vi "Move In Direction.vi"(7 "move toward? (T)":bool=TRUE, 10 "direction options":T1[](array[typedef])=[enum."NW", enum."N", enum."NE", enum."E", enum."SE", enum."S", enum."SW", enum."W"], 11 "goal angle (deg)":dbl) -> (2 "ordered directions":T1[](array[typedef]), 3 "best direction":T1)   [LabVIEW 2020, in "DS Square.lvlib"]
uses:
  DS Square.lvlib
  Type Defs/Direction Enum.ctl
  <vilib>/Analysis/baseanly.llb/Real Dot Product.vi
  <vilib>/Analysis/NI_AALBase.lvlib
  Type Defs/SB Type Defs.lvlib
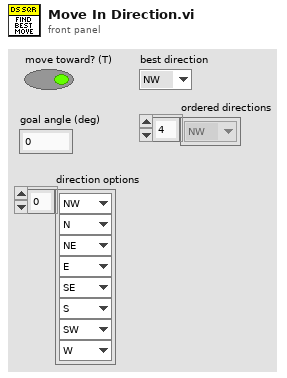
[diagram p1: front panel]
types:
  T1 = typedef "SB Type Defs.lvlib/Direction Enum.ctl" = enum16{"NW", "N", "NE", "E", "SE", "S", "SW", "W"}
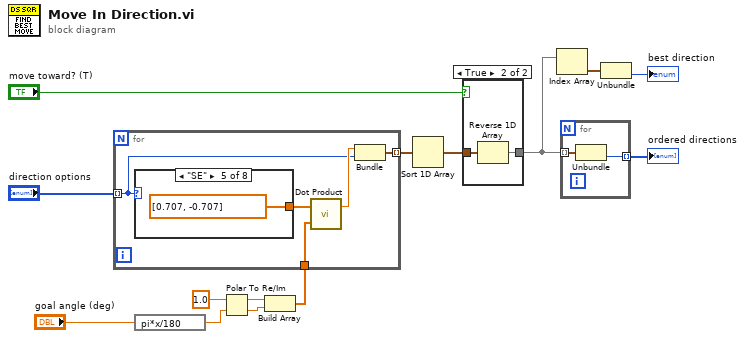
[diagram p0: block diagram]
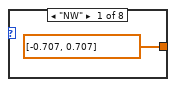
[diagram p3: hidden frame]
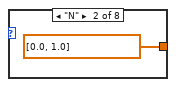
[diagram p4: hidden frame]
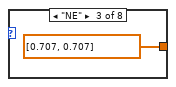
[diagram p5: hidden frame]
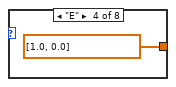
[diagram p6: hidden frame]
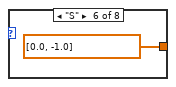
[diagram p7: hidden frame]
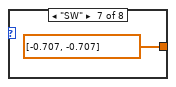
[diagram p8: hidden frame]
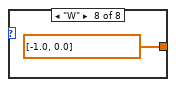
[diagram p9: hidden frame]
diagram:
  n1 = expression code="pi*x/180"("goal angle (deg)") -> (w2:dbl)
  n2 = Polar To Re/Im(2:w2, 3:1.0 ("r")) -> (0:w12:dbl, 1:w13:dbl)
  n3 = Build Array(w13, w12) -> (w11:dbl[])
  n4 = for {
    tunnel: "direction options" -> [w16] mode=indexing
    tunnel: w11 -> [w18]
    tunnel: [w15] -> w10 mode=indexing
    n5 = case shown="\"SE\"" w16 {
      tunnel: [dbl[] [-0.707, 0.707] ("X Vector") dbl[] [0.0, 1.0] ("X Vector") dbl[] [0.707, 0.707] ("X Vector") dbl[] [1.0, 0.0] ("X Vector") dbl[] [0.707, -0.707] ("X Vector") dbl[] [0.0, -1.0] ("X Vector") dbl[] [-0.707, -0.707] ("X Vector") dbl[] [-1.0, 0.0] ("X Vector")] -> w19
      frame "NW" {
      }
      frame "N" {
      }
      frame "NE" {
      }
      frame "E" {
      }
      frame "SE" {
      }
      frame "S" {
      }
      frame "SW" {
      }
      frame "W" {
      }
    }
    n6 = call-poly <vilib>:"Dot Product.vi"("Y Vector"=w18, "X Vector"=w19) -> ("X * Y"=w17:dbl)  [unwired: 1 out]
    n7 = Bundle("X * Y"=w17, "Direction"=w16) -> (w15:cluster{"X * Y":dbl, "Direction":T1})  [unwired: 1 in]
  }
  n8 = Sort 1D Array(array=w10) -> (sorted array=w9:cluster{"X * Y":dbl, "Direction":T1}[])
  n9 = case shown="True" "move toward? (T)" {
    tunnel: w9 -> [w28 w30]
    tunnel: [w28 w29] -> w6
    frame False {
    }
    frame True {
      n10 = Reverse 1D Array(array=w30) -> (reversed array=w29:cluster{"X * Y":dbl, "Direction":T1}[])
    }
  }
  n11 = Index Array(array=w6) -> (element=w5:cluster{"X * Y":dbl, "Direction":T1})  [unwired: 1 in]
  n12 = for {
    tunnel: w6 -> [w32] mode=indexing
    tunnel: [w31] -> w8 mode=indexing
    n13 = Unbundle(w32) -> ("Direction"=w31:T1)  [unwired: 1 out]
  }
  "ordered directions" <- w8
  n14 = Unbundle(w5) -> ("Direction"=→"best direction":T1)  [unwired: 1 out]
